vi "RampManipulator.vi"(7 "speed":dbl, 8 "rampManipDown":bool, 9 "rampManipUp":bool) -> (3 "rampMotorValue":dbl)   [LabVIEW 2012]
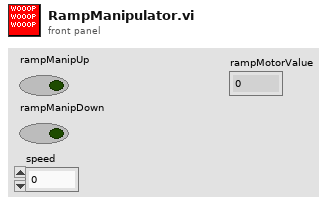
[diagram p1: front panel]
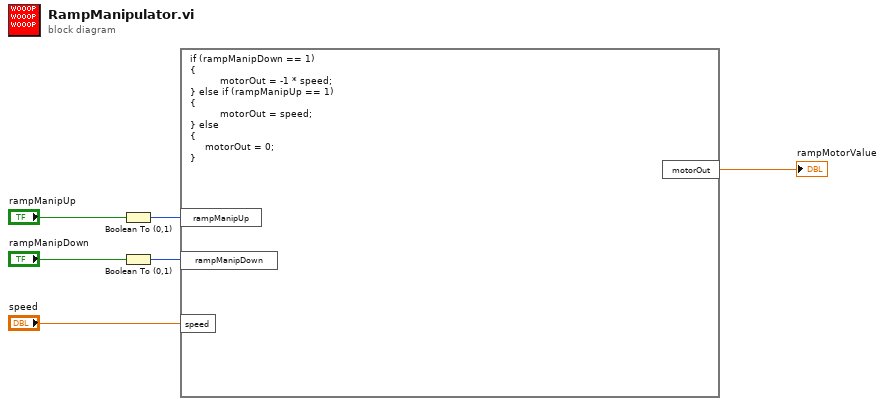
[diagram p0: block diagram]
diagram:
  n1 = Boolean To (0,1)(Boolean="rampManipUp") -> (0, 1=w3:i16)
  n2 = Boolean To (0,1)(Boolean="rampManipDown") -> (0, 1=w6:i16)
  n3 = formula code="if (rampManipDown == 1)\n{\n          motorOut = -1 * speed;\n} else if (rampManipUp == 1)\n{\n          motorOut = speed;\n} else\n{\n     motorOut = 0;\n}"("rampManipDown"=w6, "rampManipUp"=w3, "speed"="speed") -> ("motorOut"=→"rampMotorValue":dbl)
